vi "超标留样启动命令.vi"   [LabVIEW 2016]
types:
  T1 = enum16{"德润DR803M", "德润DR803L", "德润DR803F", "科盛超标留样"}
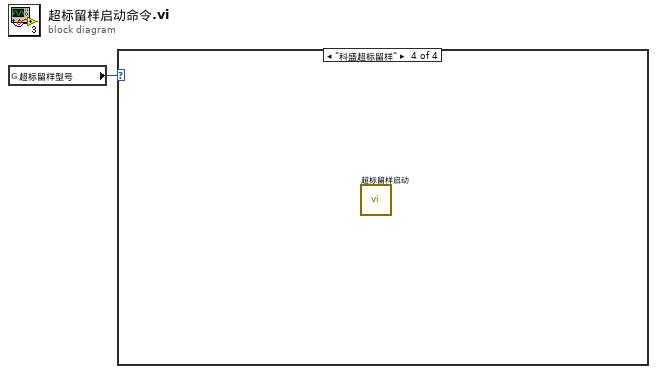
[diagram p0: block diagram]
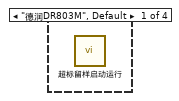
[diagram p2: hidden frame]
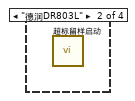
[diagram p3: hidden frame]
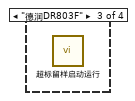
[diagram p4: hidden frame]
diagram:
  n1 = global read "断电保存全局.vi" "超标留样型号"() -> (w1:T1)
  n2 = case shown="\"科盛超标留样\"" w1 {
    frame "德润DR803M", Default {
      n3 = call "超标留样启动运行.vi"() -> ()  [unwired: 11 in, 1 out]
    }
    frame "德润DR803L" {
      n4 = call "超标留样启动.vi"() -> ()  [unwired: 11 in, 1 out]
    }
    frame "德润DR803F" {
      n5 = call "超标留样启动运行.vi"() -> ()  [unwired: 11 in, 1 out]
    }
    frame "科盛超标留样" {
      n6 = call "超标留样启动.vi"() -> ()  [unwired: 11 in, 1 out]
    }
  }
